vi "Camera Angle Calc.vi"(1 "Front Camera In":T1) -> (0 "Front Camera Out":T1)   [LabVIEW 2013]
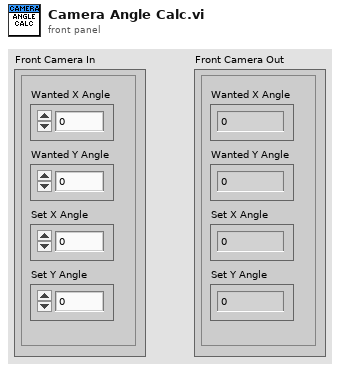
[diagram p1: front panel]
types:
  T1 = cluster{"Wanted X Angle":dbl, "Wanted Y Angle ":dbl, "Set X Angle":dbl, "Set Y Angle ":dbl}
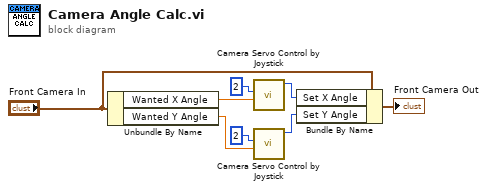
[diagram p0: block diagram]
diagram:
  n1 = Unbundle By Name("Front Camera In") -> ("Wanted X Angle"=w5:dbl, "Wanted Y Angle"=w1:dbl)
  n2 = call "Camera Servo Control by Joystick.vi"("axis control"=w5, "max jump angle"=2) -> ("angle set"=w4:i32)  [unwired: 9 in]
  n3 = call "Camera Servo Control by Joystick.vi"("axis control"=w1, "max jump angle"=2) -> ("angle set"=w2:i32)  [unwired: 9 in]
  n4 = Bundle By Name(cluster="Front Camera In", "Set X Angle"=w4, "Set Y Angle"=w2) -> (→"Front Camera Out":T1)
